vi "Wait for OPC.vi"(8 "error in (no error)":errorcluster, 10 "Time Target (s)":dbl=90.0 format="%#_13g", 11 "SpecA_MXA.lvclass.In":refnum<class "SpecA_MXA.lvclass">) -> (0 "error out":errorcluster, 2 "OPC?":bool, 3 "SpecA_MXA.lvclass.Out":refnum<class "SpecA_MXA.lvclass">)   [LabVIEW 2014, in "SpecA_MXA.lvclass"]
doc: "Waits for the current sweep to finish. You can use this VI after Initiate VI and before Fetch Trace VI.\n\n<B>Note:</B> \n\nUse this VI only with other low-level VIs. The high-level VIs automatically incorporate this functionality. This VI does not check the instrument status."
uses:
  SpecA_MXA.lvclass
  SpecA_MXA.lvclass/SpecA_MXA.ctl
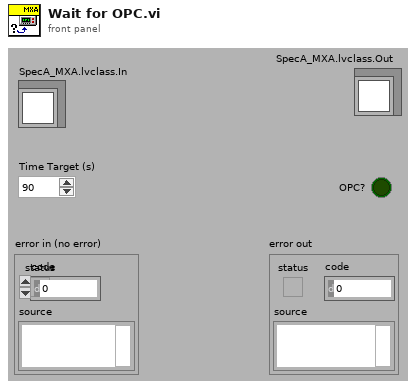
[diagram p1: front panel]
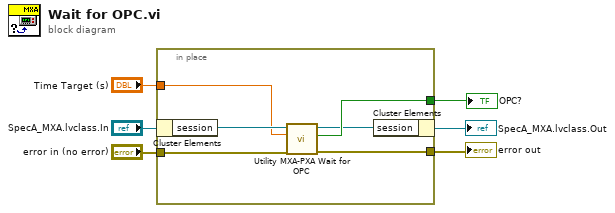
[diagram p0: block diagram]
diagram:
  n1 = in-place {
    in-place-border: "error in (no error)" -> [w12]
    in-place-border: [w10] -> w3
    in-place-border: [w8] -> w2
    in-place-border: "Time Target (s)" -> [w9]
    n2 = in-place-cluster #1("SpecA_MXA.lvclass.In") -> ("session"=w11:refnum<visa-resource-name>)
    n3 = call "Utility MXA-PXA Wait for OPC.vi"("Wait (s)"=w9, "Error In"=w12, "VISA Resource In"=w11) -> ("Error Out"=w10:errorcluster, "OPC?"=w8:bool, "VISA Resource Out"=w7:refnum<visa-resource-name>)  [unwired: 3 in, 1 out]
    n4 = in-place-cluster #1("session"=w7) -> (→"SpecA_MXA.lvclass.Out":refnum<class "SpecA_MXA.lvclass">)
  }
  "error out" <- w3
  "OPC?" <- w2
